vi "LUT_2PlayerGameMap.vi"() -> (0 "Init Data Out":u8[](array[numeric]))   [LabVIEW 2018]
uses:
  TypDefs/Tile_Enum.ctl
panel:
  in  "GameMap":T1[][](array[typedef])=[[enum."Wall_UpperLeftCorner", enum."Wall_Horizontal", enum."Wall_Horizontal", enum."Wall_Horizontal", enum."Wall_Horizontal", enum."Wall_Horizontal", enum."Wall_Horizontal", enum."Wall_Horizontal", enum."Wall_Horizontal", enum."Wall_Horizontal", enum."Wall_Horizontal", enum."Wall_Horizontal", enum."Wall_Horizontal", enum."Wall_Horizontal", enum."Wall_Horizontal", enum."Wall_Horizontal", enum."Wall_Horizontal", enum."Wall_Horizontal", enum."Wall_Horizontal", enum."Wall_Horizontal", enum."Wall_Horizontal", enum."Wall_Horizontal", enum."Wall_Horizontal", enum."Wall_Horizontal", enum."Wall_Horizontal", enum."Wall_Horizontal", enum."Wall_Horizontal", enum."Wall_Horizontal", enum."Wall_Horizontal", enum."Wall_Horizontal", enum."Wall_Horizontal", enum."Wall_UpperRightCorner"], [enum."Wall_Vertical", enum."Empty", enum."Empty", enum."Empty", enum."Empty", enum."Empty", enum."Empty", enum."Empty", enum."Empty", enum."Empty", enum."Empty", enum."Empty", enum."Empty", enum."Empty", enum."Empty", enum."Empty", enum."Empty", enum."Empty", enum."Empty", enum."Empty", enum."Empty", enum."Empty", enum."Empty", enum."Empty", enum."Empty", enum."Empty", enum."Empty", enum."Empty", enum."Empty", enum."Empty", enum."Empty", enum."Wall_Vertical"], [enum."Wall_Vertical", enum."Empty", enum."Empty", enum."Empty", enum."Empty", enum."Empty", enum."Empty", enum."Empty", enum."Empty", enum."Empty", enum."Empty", enum."Empty", enum."Empty", enum."Empty", enum."Empty", enum."Empty", enum."Empty", enum."Empty", enum."Empty", enum."Empty", enum."Empty", enum."Empty", enum."Empty", enum."Empty", enum."Empty", enum."Empty", enum."Empty", enum."Empty", enum."Empty", enum."Empty", enum."Empty", enum."Wall_Vertical"], [enum."Wall_Vertical", enum."Empty", enum."Empty", enum."Empty", enum."Empty", enum."Empty", enum."Empty", enum."Empty", enum."Empty", enum."Empty", enum."Empty", enum."Empty", enum."Empty", enum."Empty", enum."Empty", enum."Empty", enum."Empty", enum."Empty", enum."Empty", enum."Empty", enum."Empty", enum."Empty", enum."Empty", enum."Empty", enum."Empty", enum."Empty", enum."Empty", enum."Empty", enum."Empty", enum."Empty", enum."Empty", enum."Wall_Vertical"], [enum."Wall_Vertical", enum."Empty", enum."Empty", enum."Empty", enum."Empty", enum."Empty", enum."Empty", enum."Empty", enum."Empty", enum."Empty", enum."Empty", enum."Empty", enum."Empty", enum."Empty", enum."Empty", enum."Empty", enum."Empty", enum."Empty", enum."Empty", enum."Empty", enum."Empty", enum."Empty", enum."Empty", enum."Empty", enum."Empty", enum."Empty", enum."Empty", enum."Empty", enum."Empty", enum."Empty", enum."Empty", enum."Wall_Vertical"], [enum."Wall_Vertical", enum."Empty", enum."Empty", enum."Empty", enum."Empty", enum."Empty", enum."Empty", enum."Empty", enum."Empty", enum."Empty", enum."Empty", enum."Empty", enum."Empty", enum."Empty", enum."Empty", enum."Empty", enum."Empty", enum."Empty", enum."Empty", enum."Empty", enum."Empty", enum."Empty", enum."Empty", enum."Empty", enum."Empty", enum."Empty", enum."Empty", enum."Empty", enum."Empty", enum."Empty", enum."Empty", enum."Wall_Vertical"], [enum."Wall_Vertical", enum."Empty", enum."Empty", enum."Empty", enum."Empty", enum."Empty", enum."Empty", enum."Empty", enum."Empty", enum."Empty", enum."Empty", enum."Empty", enum."Empty", enum."Empty", enum."Empty", enum."Empty", enum."Empty", enum."Empty", enum."Empty", enum."Empty", enum."Empty", enum."Empty", enum."Empty", enum."Empty", enum."Empty", enum."Empty", enum."Empty", enum."Empty", enum."Empty", enum."Empty", enum."Empty", enum."Wall_Vertical"], [enum."Wall_Vertical", enum."Empty", enum."Empty", enum."Empty", enum."Empty", enum."Empty", enum."Empty", enum."Empty", enum."Empty", enum."Empty", enum."Empty", enum."Empty", enum."Empty", enum."Empty", enum."Empty", enum."Empty", enum."Empty", enum."Empty", enum."Empty", enum."Empty", enum."Empty", enum."Empty", enum."Empty", enum."Empty", enum."Empty", enum."Empty", enum."Empty", enum."Empty", enum."Empty", enum."Empty", enum."Empty", enum."Wall_Vertical"], [enum."Wall_Vertical", enum."Empty", enum."Empty", enum."Snake1_TailPointingLeft", enum."Snake1_Horizontal", enum."Snake1_Horizontal", enum."Snake1_Horizontal", enum."Snake1_Horizontal", enum."Snake1_Horizontal", enum."Snake1_HeadPointingRight", enum."Empty", enum."Empty", enum."Empty", enum."Empty", enum."Empty", enum."Empty", enum."Empty", enum."Empty", enum."Empty", enum."Empty", enum."Empty", enum."Empty", enum."Empty", enum."Empty", enum."Empty", enum."Empty", enum."Empty", enum."Empty", enum."Empty", enum."Empty", enum."Empty", enum."Wall_Vertical"], [enum."Wall_Vertical", enum."Empty", enum."Empty", enum."Empty", enum."Empty", enum."Empty", enum."Empty", enum."Empty", enum."Empty", enum."Empty", enum."Empty", enum."Empty", enum."Empty", enum."Empty", enum."Empty", enum."Empty", enum."Empty", enum."Empty", enum."Empty", enum."Empty", enum."Empty", enum."Empty", enum."Empty", enum."Empty", enum."Empty", enum."Empty", enum."Empty", enum."Empty", enum."Empty", enum."Empty", enum."Empty", enum."Wall_Vertical"], [enum."Wall_Vertical", enum."Empty", enum."Empty", enum."Empty", enum."Empty", enum."Empty", enum."Empty", enum."Empty", enum."Empty", enum."Empty", enum."Empty", enum."Empty", enum."Empty", enum."Empty", enum."Empty", enum."Empty", enum."Empty", enum."Empty", enum."Empty", enum."Empty", enum."Empty", enum."Empty", enum."Empty", enum."Empty", enum."Empty", enum."Empty", enum."Empty", enum."Empty", enum."Empty", enum."Empty", enum."Empty", enum."Wall_Vertical"], [enum."Wall_Vertical", enum."Empty", enum."Empty", enum."Empty", enum."Empty", enum."Empty", enum."Empty", enum."Empty", enum."Empty", enum."Empty", enum."Empty", enum."Empty", enum."Empty", enum."Empty", enum."Empty", enum."Empty", enum."Empty", enum."Empty", enum."Empty", enum."Empty", enum."Empty", enum."Empty", enum."Empty", enum."Empty", enum."Empty", enum."Empty", enum."Empty", enum."Empty", enum."Empty", enum."Empty", enum."Empty", enum."Wall_Vertical"], [enum."Wall_Vertical", enum."Empty", enum."Empty", enum."Empty", enum."Empty", enum."Empty", enum."Empty", enum."Empty", enum."Empty", enum."Empty", enum."Empty", enum."Empty", enum."Empty", enum."Empty", enum."Empty", enum."Empty", enum."Empty", enum."Empty", enum."Empty", enum."Empty", enum."Empty", enum."Empty", enum."Empty", enum."Empty", enum."Empty", enum."Empty", enum."Empty", enum."Empty", enum."Empty", enum."Empty", enum."Empty", enum."Wall_Vertical"], [enum."Wall_Vertical", enum."Empty", enum."Empty", enum."Empty", enum."Empty", enum."Empty", enum."Empty", enum."Empty", enum."Empty", enum."Empty", enum."Empty", enum."Empty", enum."Empty", enum."Empty", enum."Empty", enum."Empty", enum."Empty", enum."Empty", enum."Empty", enum."Empty", enum."Empty", enum."Empty", enum."Empty", enum."Empty", enum."Empty", enum."Empty", enum."Empty", enum."Empty", enum."Empty", enum."Empty", enum."Empty", enum."Wall_Vertical"], [enum."Wall_Vertical", enum."Empty", enum."Empty", enum."Empty", enum."Empty", enum."Empty", enum."Empty", enum."Empty", enum."Empty", enum."Empty", enum."Empty", enum."Empty", enum."Empty", enum."Empty", enum."Empty", enum."Empty", enum."Empty", enum."Empty", enum."Empty", enum."Empty", enum."Empty", enum."Empty", enum."Empty", enum."Empty", enum."Empty", enum."Empty", enum."Empty", enum."Empty", enum."Empty", enum."Empty", enum."Empty", enum."Wall_Vertical"], [enum."Wall_Vertical", enum."Empty", enum."Empty", enum."Empty", enum."Empty", enum."Empty", enum."Empty", enum."Empty", enum."Empty", enum."Empty", enum."Empty", enum."Empty", enum."Empty", enum."Empty", enum."Empty", enum."Empty", enum."Empty", enum."Empty", enum."Empty", enum."Empty", enum."Empty", enum."Empty", enum."Snake2_HeadPointingLeft", enum."Snake2_Horizontal", enum."Snake2_Horizontal", enum."Snake2_Horizontal", enum."Snake2_Horizontal", enum."Snake2_Horizontal", enum."Snake2_TailPointingRight", enum."Empty", enum."Empty", enum."Wall_Vertical"], [enum."Wall_Vertical", enum."Empty", enum."Empty", enum."Empty", enum."Empty", enum."Empty", enum."Empty", enum."Empty", enum."Empty", enum."Empty", enum."Empty", enum."Empty", enum."Empty", enum."Empty", enum."Empty", enum."Empty", enum."Empty", enum."Empty", enum."Empty", enum."Empty", enum."Empty", enum."Empty", enum."Empty", enum."Empty", enum."Empty", enum."Empty", enum."Empty", enum."Empty", enum."Empty", enum."Empty", enum."Empty", enum."Wall_Vertical"], [enum."Wall_Vertical", enum."Empty", enum."Empty", enum."Empty", enum."Empty", enum."Empty", enum."Empty", enum."Empty", enum."Empty", enum."Empty", enum."Empty", enum."Empty", enum."Empty", enum."Empty", enum."Empty", enum."Empty", enum."Empty", enum."Empty", enum."Empty", enum."Empty", enum."Empty", enum."Empty", enum."Empty", enum."Empty", enum."Empty", enum."Empty", enum."Empty", enum."Empty", enum."Empty", enum."Empty", enum."Empty", enum."Wall_Vertical"], [enum."Wall_Vertical", enum."Empty", enum."Empty", enum."Empty", enum."Empty", enum."Empty", enum."Empty", enum."Empty", enum."Empty", enum."Empty", enum."Empty", enum."Empty", enum."Empty", enum."Empty", enum."Empty", enum."Empty", enum."Empty", enum."Empty", enum."Empty", enum."Empty", enum."Empty", enum."Empty", enum."Empty", enum."Empty", enum."Empty", enum."Empty", enum."Empty", enum."Empty", enum."Empty", enum."Empty", enum."Empty", enum."Wall_Vertical"], [enum."Wall_Vertical", enum."Empty", enum."Empty", enum."Empty", enum."Empty", enum."Empty", enum."Empty", enum."Empty", enum."Empty", enum."Empty", enum."Empty", enum."Empty", enum."Empty", enum."Empty", enum."Empty", enum."Empty", enum."Empty", enum."Empty", enum."Empty", enum."Empty", enum."Empty", enum."Empty", enum."Empty", enum."Empty", enum."Empty", enum."Empty", enum."Empty", enum."Empty", enum."Empty", enum."Empty", enum."Empty", enum."Wall_Vertical"], [enum."Wall_Vertical", enum."Empty", enum."Empty", enum."Empty", enum."Empty", enum."Empty", enum."Empty", enum."Empty", enum."Empty", enum."Empty", enum."Empty", enum."Empty", enum."Empty", enum."Empty", enum."Empty", enum."Empty", enum."Empty", enum."Empty", enum."Empty", enum."Empty", enum."Empty", enum."Empty", enum."Empty", enum."Empty", enum."Empty", enum."Empty", enum."Empty", enum."Empty", enum."Empty", enum."Empty", enum."Empty", enum."Wall_Vertical"], [enum."Wall_Vertical", enum."Empty", enum."Empty", enum."Empty", enum."Empty", enum."Empty", enum."Empty", enum."Empty", enum."Empty", enum."Empty", enum."Empty", enum."Empty", enum."Empty", enum."Empty", enum."Empty", enum."Empty", enum."Empty", enum."Empty", enum."Empty", enum."Empty", enum."Empty", enum."Empty", enum."Empty", enum."Empty", enum."Empty", enum."Empty", enum."Empty", enum."Empty", enum."Empty", enum."Empty", enum."Empty", enum."Wall_Vertical"], [enum."Wall_Vertical", enum."Empty", enum."Empty", enum."Empty", enum."Empty", enum."Empty", enum."Empty", enum."Empty", enum."Empty", enum."Empty", enum."Empty", enum."Empty", enum."Empty", enum."Empty", enum."Empty", enum."Empty", enum."Empty", enum."Empty", enum."Empty", enum."Empty", enum."Empty", enum."Empty", enum."Empty", enum."Empty", enum."Empty", enum."Empty", enum."Empty", enum."Empty", enum."Empty", enum."Empty", enum."Empty", enum."Wall_Vertical"], [enum."Wall_LowerLeftCorner", enum."Wall_Horizontal", enum."Wall_Horizontal", enum."Wall_Horizontal", enum."Wall_Horizontal", enum."Wall_Horizontal", enum."Wall_Horizontal", enum."Wall_Horizontal", enum."Wall_Horizontal", enum."Wall_Horizontal", enum."Wall_Horizontal", enum."Wall_Horizontal", enum."Wall_Horizontal", enum."Wall_Horizontal", enum."Wall_Horizontal", enum."Wall_Horizontal", enum."Wall_Horizontal", enum."Wall_Horizontal", enum."Wall_Horizontal", enum."Wall_Horizontal", enum."Wall_Horizontal", enum."Wall_Horizontal", enum."Wall_Horizontal", enum."Wall_Horizontal", enum."Wall_Horizontal", enum."Wall_Horizontal", enum."Wall_Horizontal", enum."Wall_Horizontal", enum."Wall_Horizontal", enum."Wall_Horizontal", enum."Wall_Horizontal", enum."Wall_LowerRightCorner"]]
  # "For Initialization VI requirements and help, please read directions located on Block Diagram."
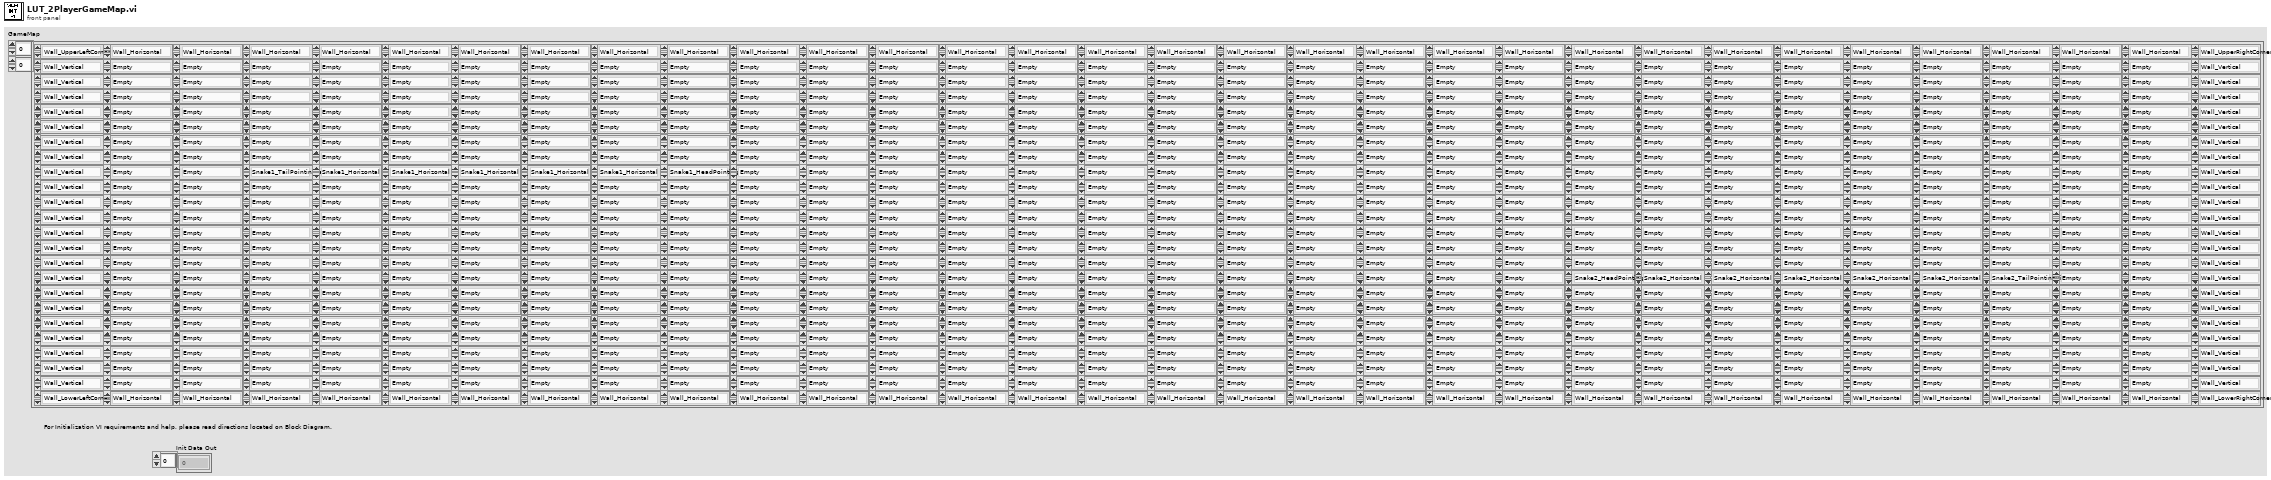
[diagram p1: front panel]
types:
  T1 = typedef "Tile_Enum.ctl" = enum8{"Empty", "Snake1_HeadPointingUp", "Snake1_HeadPointingDown", "Snake1_HeadPointingLeft", "Snake1_HeadPointingRight", "Snake1_DeadPointingUp", "Snake1_DeadPointingDown", "Snake1_DeadPointingLeft", "Snake1_DeadPointingRight", "Snake1_TailPointingUp", "Snake1_TailPointingDown", "Snake1_TailPointingLeft", "Snake1_TailPointingRight", "Snake1_Horizontal", "Snake1_Vertical", "Snake1_UpperLeftCorner", "Snake1_UpperRightCorner", "Snake1_LowerLeftCorner", "Snake1_LowerRightCorner", "Snake2_HeadPointingUp", "Snake2_HeadPointingDown", "Snake2_HeadPointingLeft", "Snake2_HeadPointingRight", "Snake2_DeadPointingUp", "Snake2_DeadPointingDown", "Snake2_DeadPointingLeft", "Snake2_DeadPointingRight", "Snake2_TailPointingUp", "Snake2_TailPointingDown", "Snake2_TailPointingLeft", "Snake2_TailPointingRight", "Snake2_Horizontal", "Snake2_Vertical", "Snake2_UpperLeftCorner", "Snake2_UpperRightCorner", "Snake2_LowerLeftCorner", "Snake2_LowerRightCorner", "Wall_Horizontal", "Wall_Vertical", "Wall_UpperLeftCorner", "Wall_UpperRightCorner", "Wall_LowerLeftCorner", "Wall_LowerRightCorner", "Pickup_SpeedUp", "Pickup_SlowDown", "Pickup_Banana", "Pickup_Grapes", "Pickup_Apple"}
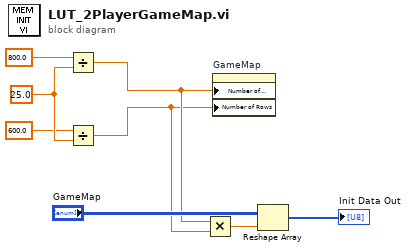
[diagram p0: block diagram]
diagram:
  w7 = 25.0 ("y")
  n1 = Divide(x=800.0, y=w7) -> (x/y=w4:dbl)
  n2 = Divide(x=600.0, y=w7) -> (x/y=w3:dbl)
  n3 = Multiply(x=w4, y=w3) -> (x*y=w2:dbl)
  n4 = property on="GameMap" class="Arr (strict)"("Number of Columns"=w4, "Number of Rows"=w3) -> ()  [unwired: 2 in, 2 out]
  n5 = Reshape Array("GameMap", w2) -> (→"Init Data Out":T1[])
